vi "Read Semaphore.vi"(8 "error in (no error)":errorcluster, 11 "Future in":refnum<class "Future.lvclass">) -> (0 "error out":errorcluster, 2 "semaphore":T1, 3 "Future out":refnum<class "Future.lvclass">)   [LabVIEW 2017, in "Promise Future.lvlib" / "Future.lvclass"]
uses:
  Future.lvclass
  Future.lvclass/Future.ctl
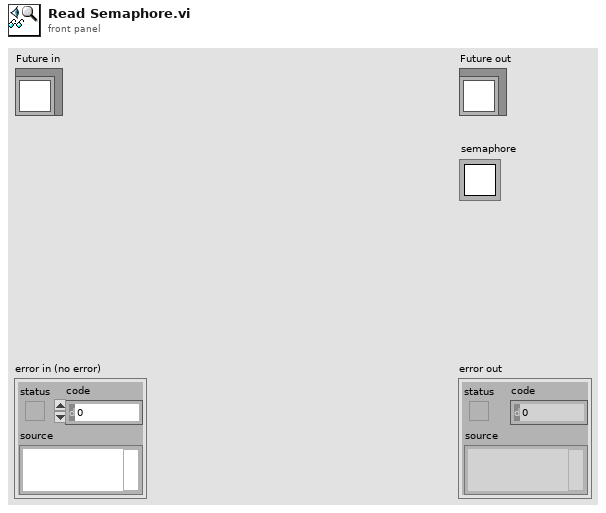
[diagram p1: front panel]
types:
  T1 = typedef "Semaphore RefNum" = refnum<k1>
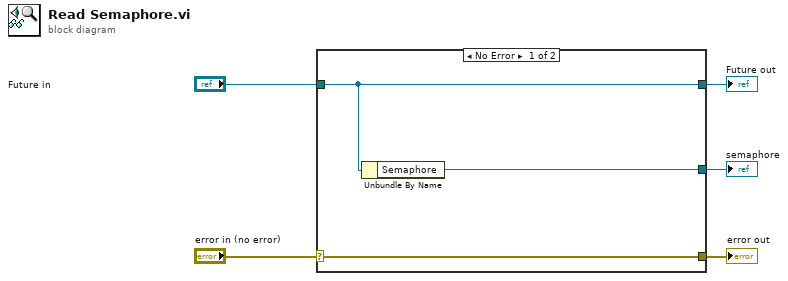
[diagram p0: block diagram]
diagram:
  n1 = case shown="No Error" "error in (no error)" {
    selector: "error in (no error)" -> [w8 w9]
    tunnel: [w8 w9] -> w4
    tunnel: [w7 w10] -> w2
    tunnel: "Future in" -> [w7 w10]
    tunnel: [w6 _] -> w1
    frame No Error {
      n2 = Unbundle By Name(w7) -> ("Semaphore"=w6:T1)
    }
    frame Error {
    }
  }
  "error out" <- w4
  "Future out" <- w2
  "semaphore" <- w1
